vi "LV_UDP_RCVR.vi"() -> ()   [LabVIEW 2020]
uses:
  <vilib>/Analysis/baseanly.llb/Mean (DBL).vi
  <vilib>/Analysis/NI_AALBase.lvlib
panel:
  out "Received Array":dbl[](array[numeric])
  out "Loop Time Mean (ms x 1000)":dbl format="%0.2f"
  in  "Number of samples":i32
  out "Loop Time (ms)":dbl
  out "Received String":string
  in  "Stop":bool
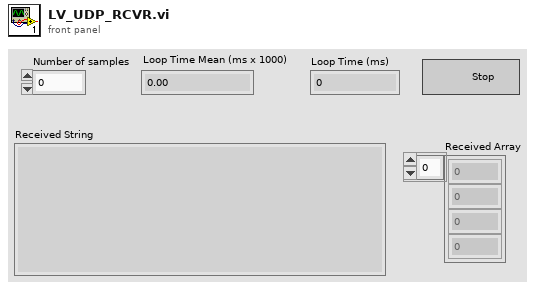
[diagram p1: front panel]
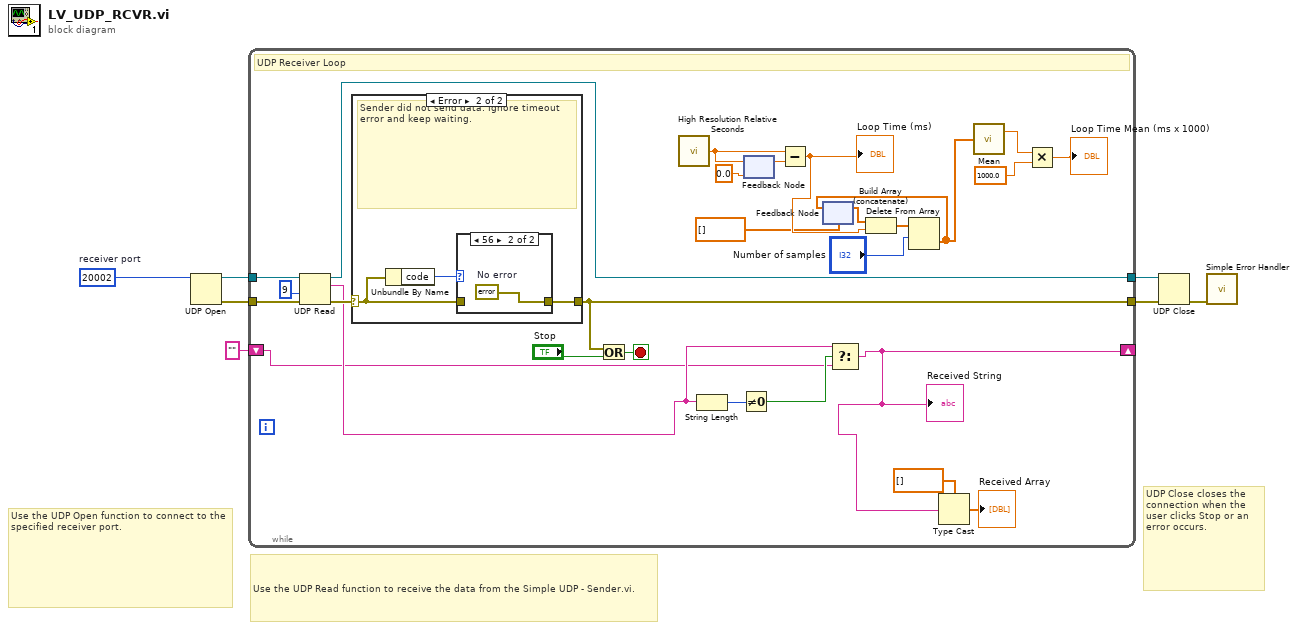
[diagram p0: block diagram]
diagram:
  w2 = u16 20002  # receiver port
  # "UDP Close closes the connection when the user clicks Stop or an error occurs."
  # "Use the UDP Open function to connect to the specified receiver port."
  # "Use the UDP Read function to receive the data from the Simple UDP - Sender.vi."
  n1 = UDP Open(11:w2) -> (port=w3:refnum<k16>, 0:w4:errorcluster)  [unwired: 4 in, 1 out]
  n2 = while {
    tunnel: w3 -> [w34]
    tunnel: [w27] -> w7
    tunnel: w4 -> [w31]
    tunnel: [w28] -> w5
    shift-right: [w9] -> _
    shift-left: "" ("data out") -> [w11]
    stop <- w32 stop-if-true
    # "UDP Receiver Loop"
    n3 = UDP Read(connection ID=w34, timeout ms (25000)=9, 8:w31) -> (data out=w12:string, error out=w29:errorcluster, 3:w27:refnum<k16>)  [unwired: 3 out]
    n4 = case shown="Error" w29 {
      selector: w29 -> [w35 w37]
      tunnel: [w35 w36] -> w28
      frame No Error {
        # "Sender sent data. Update the chart value."
      }
      frame Error {
        # "Sender did not send data. Ignore timeout error and keep waiting."
        n5 = Unbundle By Name(w37) -> ("code"=w38:i32)
        n6 = case shown="56" w38 {
          tunnel: w37 -> [w39 _]
          tunnel: [w39 w40] -> w36
          frame Default {
          }
          frame 56 {
            w40 = errorcluster {"status"=FALSE, "code"=0, "source"=""}  # No error
          }
        }
      }
    }
    n7 = Or(x=w28, y="Stop") -> (x .or. y?=w32:bool)
    n8 = call <vilib>:"High Resolution Relative Seconds.vi"() -> ("relative seconds"=w24:dbl)
    n9 = String Length(string=w12) -> (length=w14:i32)
    n10 = Not Equal To 0?(x=w14) -> (x != 0?=w13:bool)
    n11 = feedback-in #1(w24) -> ()
    n12 = feedback #1(0.0 ("millisecond timer value")) -> (w26:dbl)
    n13 = Subtract(x=w24, y=w26) -> (x-y=w20:dbl)
    "Loop Time (ms)" <- w20
    n14 = feedback #2(dbl[] []) -> (w22:dbl[])
    n15 = Select(t=w12, s=w13, f=w11) -> (s? t:f=w9:string)
    "Received String" <- w9
    n16 = Build Array (concatenate)(w22, w20) -> (w21:dbl[])
    n17 = Delete From Array(array=w21, length="Number of samples") -> (deleted portion=w18:dbl[])  [unwired: 1 in, 1 out]
    n18 = feedback-in #2(w18) -> ()
    n19 = Type Cast(type=dbl[] [], x=w9) -> (*(type *) &x=→"Received Array":dbl[])
    n20 = call-poly <vilib>:"Mean.vi"("X"=w18) -> ("mean"=w17:dbl)  [unwired: 1 out]
    n21 = Multiply(x=w17, y=1000.0) -> (x*y=→"Loop Time Mean (ms x 1000)":dbl)
  }
  n22 = UDP Close(connection ID=w7, 8:w5) -> (error out=w6:errorcluster)  [unwired: 1 out]
  n23 = call <vilib>:"Simple Error Handler.vi"("error in (no error)"=w6) -> ()  [unwired: 1 in, 8 out]
